vi "Log_RT_1.vi"() -> ()   [LabVIEW 2019]
panel:
  out "RW Direction of Rotation TM Hisory":string
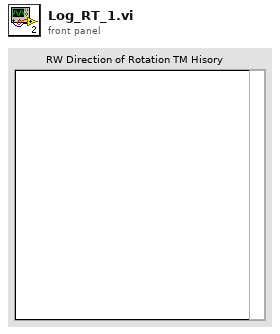
[diagram p1: front panel]
types:
  T1 = enum16{"open", "replace", "create", "open or create", "replace or create", "replace or create with confirmation"}
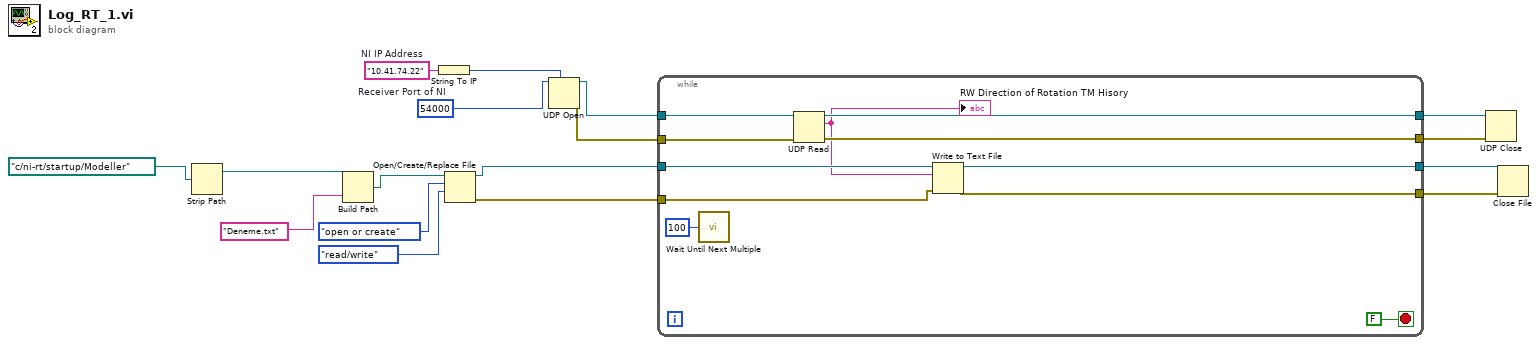
[diagram p0: block diagram]
diagram:
  w7 = "10.41.74.22"  # NI IP Address
  w6 = u16 54000  # Receiver Port of NI
  n1 = Strip Path(path=path "c:/ni-rt/startup/Modeller") -> (stripped path=w17:path)  [unwired: 1 out]
  n2 = Build Path(base path=w17, name or relative path="Deneme.txt" ("file")) -> (appended path=w16:path)
  n3 = String To IP(1:w7) -> (0:w5:u32)
  n4 = Open/Create/Replace File(file path (use dialog)=w16, operation (0:open)=T1."open or create", access (0:read/write)=enum16{"read/write", "read-only", "write-only"}."read/write") -> (refnum out=w11:refnum<file>, error out=w10:errorcluster)  [unwired: 3 in, 1 out]
  n5 = UDP Open(7:w5, 11:w6) -> (port=w4:refnum<k16>, 0:w3:errorcluster)  [unwired: 3 in, 1 out]
  n6 = while {
    tunnel: w11 -> [w27]
    tunnel: w10 -> [w26]
    tunnel: [w25] -> w9
    tunnel: [w24] -> w8
    tunnel: w4 -> [w22]
    tunnel: w3 -> [w21]
    tunnel: [w20] -> w2
    tunnel: [w19] -> w1
    stop <- FALSE stop-if-true
    n7 = call "Wait Until Next Multiple"("Count(mSec)"=u32 100) -> ()  [unwired: 1 out]
    n8 = UDP Read(connection ID=w22, 8:w21) -> (data out=w18:string, error out=w19:errorcluster, 3:w20:refnum<k16>)  [unwired: 2 in, 2 out]
    "RW Direction of Rotation TM Hisory" <- w18
    n9 = Write to Text File(file (use dialog)=w27, text=w18, error in=w26) -> (refnum out=w25:refnum<file>, error out=w24:errorcluster)  [unwired: 1 in, 1 out]
  }
  n10 = UDP Close(connection ID=w2, 8:w1) -> ()  [unwired: 2 out]
  n11 = Close File(refnum=w9, error in=w8) -> ()  [unwired: 2 out]
